vi "Unflatten Value.vi"(8 "Error In":errorcluster, 10 "Value":string, 11 "2D Path In":refnum<class "2D Path.lvclass">) -> (0 "Error Out":errorcluster, 3 "2D Path Out":refnum<class "2D Path.lvclass">)   [LabVIEW 2017, in "Tree API.lvlib" / "2D Path.lvclass"]
doc: "Dynamic dispatch interface for unflattening Tree Data classes from string."
uses:
  2D Path.lvclass
  Tree Manager/Tree.lvclass
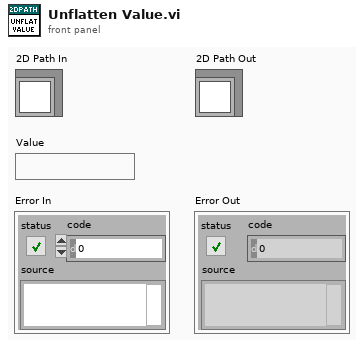
[diagram p1: front panel]
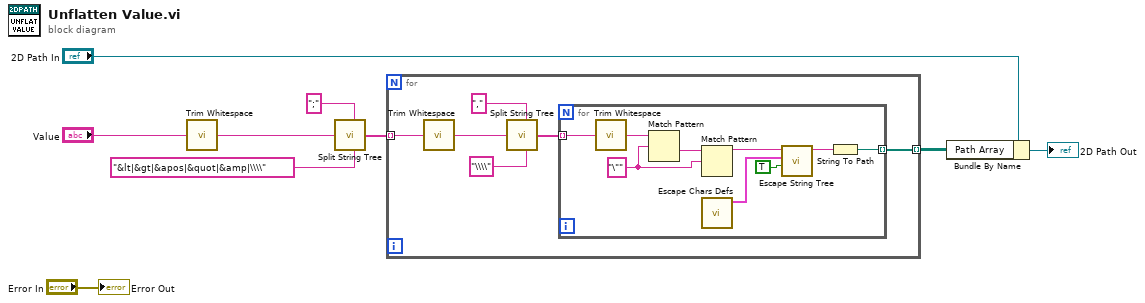
[diagram p0: block diagram]
diagram:
  n1 = call <vilib>:"Trim Whitespace.vi"("string"="Value") -> ("trimmed string"=w1:string)  [unwired: 1 in]
  n2 = call "Split String Tree.vi"("Ignore Pattern"="&lt|&gt|&apos|&quot|&amp|\\\\", "Split Pattern"=";", "Input String"=w1) -> ("Split String"=w5:string[])  [unwired: 4 in]
  n3 = for {
    tunnel: [w13] -> w9 mode=indexing
    tunnel: w5 -> [w12] mode=indexing
    n4 = call <vilib>:"Trim Whitespace.vi"("string"=w12) -> ("trimmed string"=w10:string)  [unwired: 1 in]
    n5 = call "Split String Tree.vi"("Ignore Pattern"="\\\\", "Split Pattern"=",", "Input String"=w10) -> ("Split String"=w14:string[])  [unwired: 4 in]
    n6 = for {
      tunnel: w14 -> [w23] mode=indexing
      tunnel: [w24] -> w13 mode=indexing
      w20 = "\"" ("regular expression")
      n7 = call <vilib>:"Trim Whitespace.vi"("string"=w23) -> ("trimmed string"=w21:string)  [unwired: 1 in]
      n8 = Match Pattern(string=w21, regular expression=w20) -> (after substring=w22:string)  [unwired: 1 in, 3 out]
      n9 = Match Pattern(string=w22, regular expression=w20) -> (before substring=w18:string)  [unwired: 1 in, 3 out]
      n10 = call "Escape Chars Defs.vi"() -> ("Escapes"=w19:cluster{"String":string, "Escape":string}[])  [unwired: 11 in]
      n11 = call "Escape String Tree.vi"("Reverse? (False)"=TRUE, "Escapes"=w19, "String In"=w18) -> ("String Out"=w17:string)  [unwired: 8 in]
      n12 = String To Path(string=w17) -> (path=w24:path)
    }
  }
  n13 = Bundle By Name(cluster="2D Path In", "Path Array"=w9) -> (→"2D Path Out":refnum<class "2D Path.lvclass">)
  "Error Out" <- "Error In"
